vi "dfd_Sort Zeros for Minimum Phase.vi"(10 "zeros":cdb[](array[numeric])) -> (1 "zeros  in h0":cdb[](array[numeric]), 2 "zeros  in g0":cdb[](array[numeric]))   [LabVIEW 2017, in "NI_DigFilter_FilterBank.lvlib"]
uses:
  <vilib>/addons/Digital Filter Design/NI_DigFilter_FilterBank.lvlib
  <vilib>/addons/Digital Filter Design/NI_DigFilter_Design.lvlib
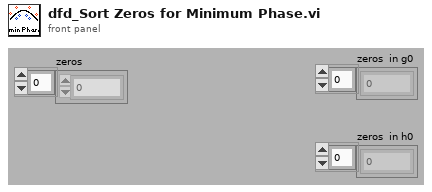
[diagram p1: front panel]
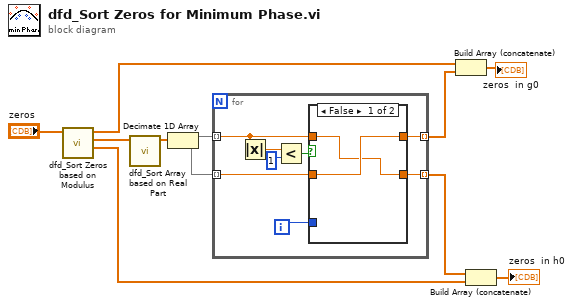
[diagram p0: block diagram]
diagram:
  n1 = call <vilib>:"dfd_Sort Zeros based on Modulus.vi"("zeros"="zeros") -> (">1"=w9:cdb[], "=1"=w5:cdb[], "<1"=w10:cdb[])  [unwired: 8 in]
  n2 = call <vilib>:"dfd_Sort Array based on Real Part.vi"("input array"=w5) -> ("sorted array"=w4:cdb[])  [unwired: 9 in, 1 out]
  n3 = Decimate 1D Array(w4) -> (w3:cdb[], w11:cdb[])
  n4 = for {
    tunnel: w3 -> [w16] mode=indexing
    tunnel: w11 -> [w14] mode=indexing
    tunnel: [w13] -> w2 mode=indexing
    tunnel: [w12] -> w1 mode=indexing
    i -> [w17]
    n5 = Absolute Value(x=w16) -> (abs(x)=w15:dbl)
    n6 = Less?(x=w15, y=1) -> (x < y?=w18:bool)
    n7 = case shown="False" w18 {
      tunnel: [w21 w23] -> w13
      tunnel: w14 -> [w21 w22]
      tunnel: [w20 w22] -> w12
      tunnel: w17 -> [_ _]
      tunnel: w16 -> [w20 w23]
      frame False {
      }
      frame True {
      }
    }
  }
  n8 = Build Array (concatenate)(w10, w2) -> (→"zeros  in g0":cdb[])
  n9 = Build Array (concatenate)(w1, w9) -> (→"zeros  in h0":cdb[])
